vi "Init Unmapped Nodes Tab.vi"(8 "error in (no error)":errorcluster, 11 "Loop Data in":T1) -> (0 "error out":errorcluster)   [LabVIEW 2016, in "System Mapping Tool.lvlib"]
uses:
  System Mapping Tool.lvlib
  TypeDefs/Loop Data.ctl
  TypeDefs/UI Refs.ctl
  NationalInstruments.VeriStand.SystemDefinitionAPI
  NationalInstruments.VeriStand.SystemStorageUI
  <vilib>/Utility/miscctls.llb/LVRowAndColumnTypeDef.ctl
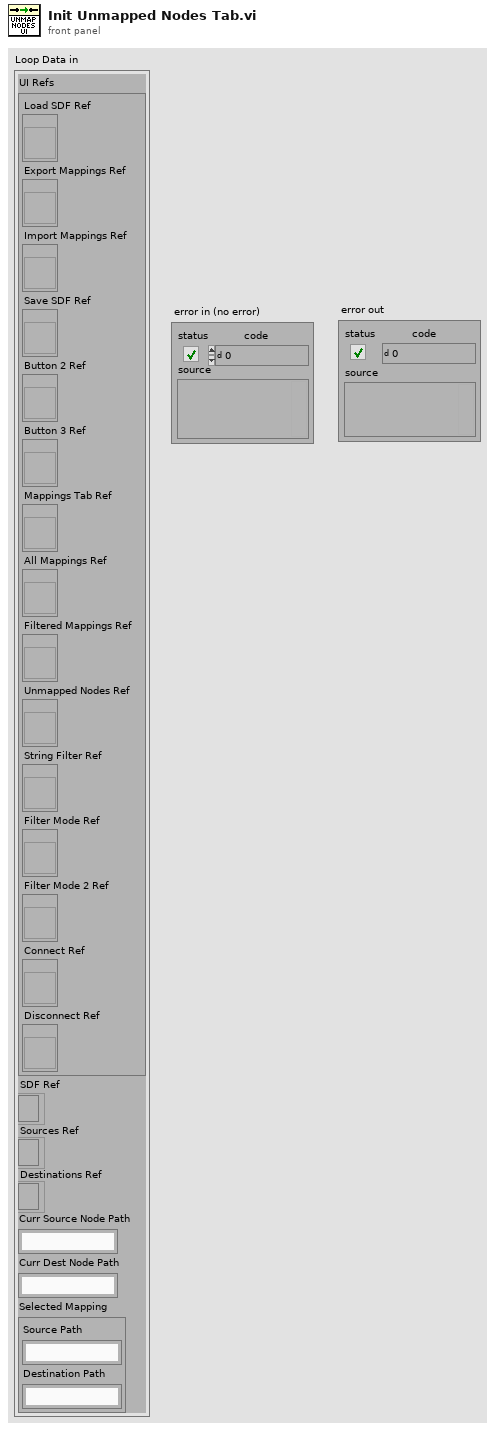
[diagram p1: front panel]
types:
  T1 = typedef "System Mapping Tool.lvlib/Loop Data.ctl" = cluster{"UI Refs":T2, "SDF Ref":refnum<k24>, "Sources Ref":refnum<k24>, "Destinations Ref":refnum<k24>, "Curr Source Node Path":string, "Curr Dest Node Path":string, "Selected Mapping":cluster{"Source Path":string, "Destination Path":string}}
  T2 = typedef "System Mapping Tool.lvlib/UI Refs.ctl" = cluster{"Load SDF Ref":refnum<vi>, "Export Mappings Ref":refnum<vi>, "Import Mappings Ref":refnum<vi>, "Save SDF Ref":refnum<vi>, "Button 2 Ref":refnum<vi>, "Button 3 Ref":refnum<vi>, "Mappings Tab Ref":refnum<vi>, "All Mappings Ref":refnum<vi>, "Filtered Mappings Ref":refnum<vi>, "Unmapped Nodes Ref":refnum<vi>, "String Filter Ref":refnum<vi>, "Filter Mode Ref":refnum<vi>, "Filter Mode 2 Ref":refnum<vi>, "Connect Ref":refnum<vi>, "Disconnect Ref":refnum<vi>}
  T3 = enum32{"All System Mappings", "Filtered Mappings by Node", "Unmapped Channels by Node"}
  T4 = typedef "LVRowAndColumnTypeDef.ctl" = cluster{"Row":i32, "Column":i32}
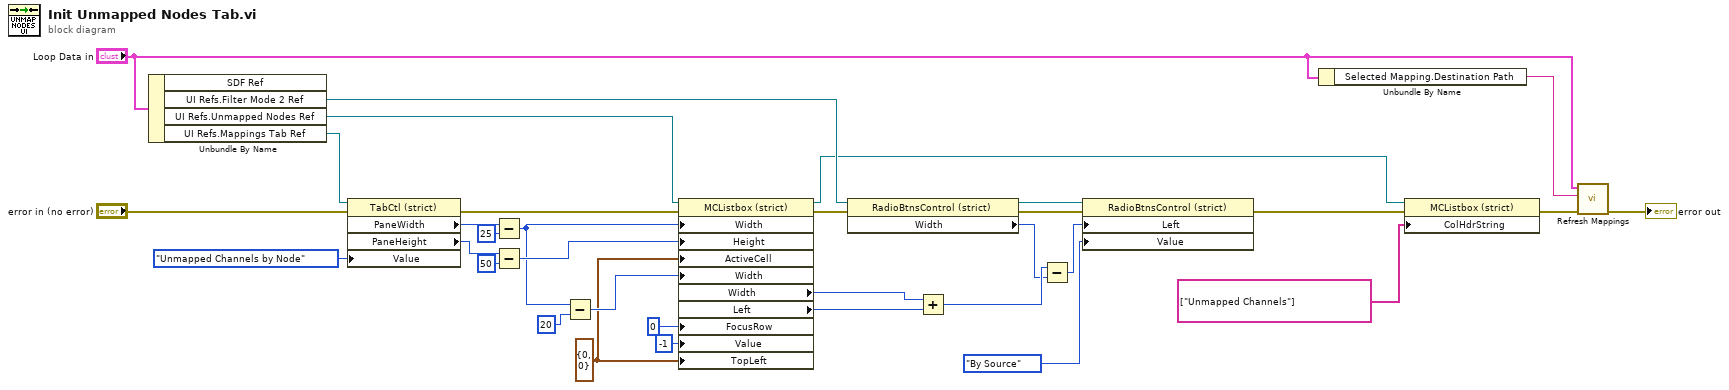
[diagram p0: block diagram]
diagram:
  w1 = T4 {"Row"=0, "Column"=0} ("Active Cell:Active Cell")
  n1 = Unbundle By Name("Loop Data in") -> ("UI Refs.Filter Mode 2 Ref"=w18:refnum<vi>, "UI Refs.Unmapped Nodes Ref"=w23:refnum<vi>, "UI Refs.Mappings Tab Ref"=w24:refnum<vi>)  [unwired: 1 out]
  n2 = property class="TabCtl (strict)"(reference=w24, error in="error in (no error)", "Value"=T3."Unmapped Channels by Node") -> (error out=w33:errorcluster, "PaneWidth"=w30:u32, "PaneHeight"=w27:u32)  [unwired: 1 out]
  n3 = Subtract(x=w30, y=u32 25) -> (x-y=w25:u32)
  n4 = Subtract(x=w27, y=u32 50) -> (x-y=w26:u32)
  n5 = Subtract(x=w25, y=u32 20) -> (x-y=w31:u32)
  n6 = property class="MCListbox (strict)"(reference=w23, error in=w33, "Width"=w25, "Height"=w26, "ActiveCell"=w1, "Width"=w31, "FocusRow"=0 ("Focus Row"), "Value"=-1, "TopLeft"=w1) -> (reference out=w11:refnum<vi>, error out=w16:errorcluster, "Width"=w20:u32, "Left"=w21:i32)
  n7 = property class="RadioBtnsControl (strict)"(reference=w18, error in=w16) -> (reference out=w17:refnum<vi>, error out=w19:errorcluster, "Width"=w14:u32)
  n8 = Add(x=w20, y=w21) -> (x+y=w15:u32)
  n9 = Subtract(x=w15, y=w14) -> (x-y=w13:u32)
  n10 = property class="RadioBtnsControl (strict)"(reference=w17, error in=w19, "Left"=w13, "Value"=enum32{"By Source", "By Destination"}."By Source") -> (error out=w8:errorcluster)  [unwired: 1 out]
  n11 = Unbundle By Name("Loop Data in") -> ("Selected Mapping.Destination Path"=w5:string)
  n12 = property class="MCListbox (strict)"(reference=w11, error in=w8, "ColHdrString"=string[] ["Unmapped Channels"] ("Row Header Strings[]")) -> (error out=w12:errorcluster)  [unwired: 1 out]
  n13 = call "Refresh Mappings.vi"("error in (no error)"=w12, "Destination to Highlight"=w5, "Loop Data"="Loop Data in") -> ("error out"=→"error out":errorcluster)  [unwired: 8 in]
